vi "Stroke Calibration Report.vi"(8 "error in (no error)":errorcluster, 9 "measured_value":dbl, 10 "operator_name":string="Kiran", 11 "Instrument_serial Number":string="021099") -> (0 "error out":errorcluster, 3 "return value":string)   [LabVIEW 2025]
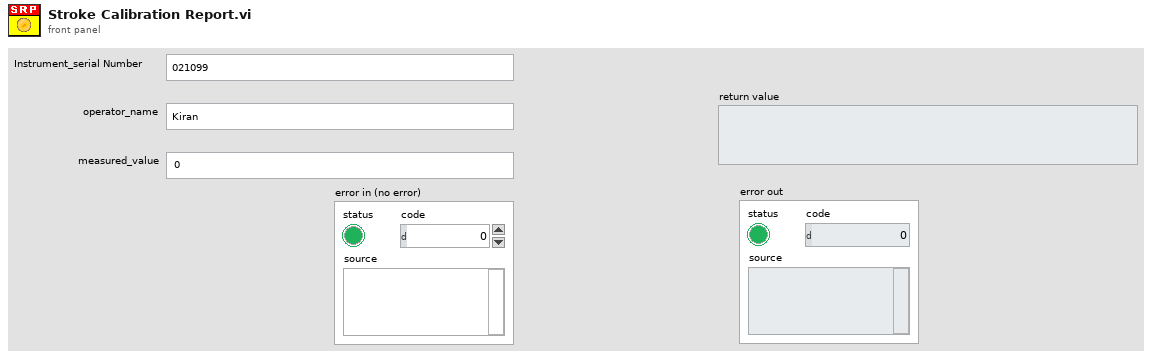
[diagram p1: front panel]
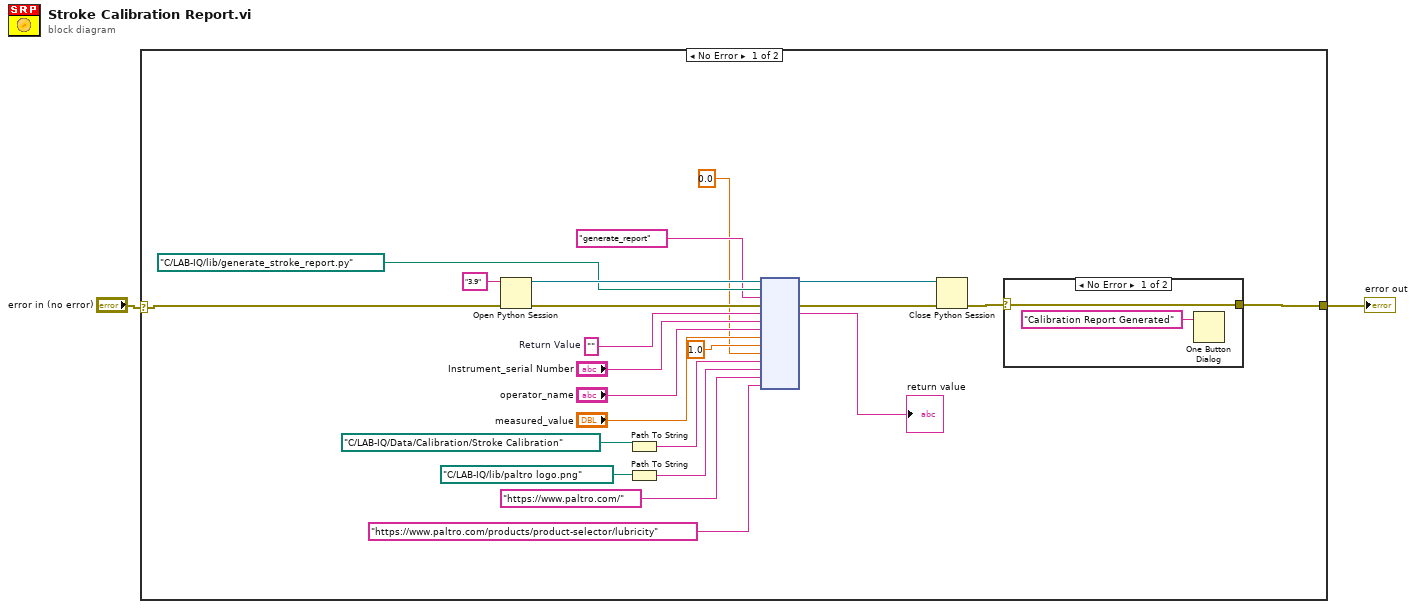
[diagram p0: block diagram]
diagram:
  n1 = case shown="No Error" "error in (no error)" {
    selector: "error in (no error)" -> [w5 _]
    tunnel: [w3 _] -> w2
    frame No Error {
      w20 = ""  # Return Value
      n2 = Open Python Session(python version="3.9" ("Python version"), 3:w5) -> (session out=w24:refnum<k35>, error out=w23:errorcluster)  [unwired: 1 in]
      n3 = Path To String(path=path "C:/LAB-IQ/Data/Calibration/Stroke Calibration" ("output_dir")) -> (string=w8:string)
      n4 = Path To String(path=path "C:/LAB-IQ/lib/paltro logo.png" ("logo_path")) -> (string=w9:string)
      n5 = node(w24, path "C:/LAB-IQ/lib/generate_stroke_report.py" ("Python path"), "generate_report" ("function name"), w23, w20, "Instrument_serial Number", "operator_name", "measured_value", 1.0 ("measured_value"), 0.0 ("measured_value"), w8, w9, "https://www.paltro.com/" ("logo_link_url"), "https://www.paltro.com/products/product-selector/lubricity" ("footer_link_url")) -> (w12:refnum<k35>, w13:errorcluster, →"return value":string)  [unwired: 9 in, 2 out]
      n6 = Close Python Session(session in=w12, error in=w13) -> (11:w4:errorcluster)
      n7 = case shown="No Error" w4 {
        selector: w4 -> [w27 _]
        tunnel: [w27 _] -> w3
        frame No Error {
          n8 = One Button Dialog(message="Calibration Report Generated") -> ()  [unwired: 1 in, 1 out]
        }
        frame Error {
        }
      }
    }
    frame Error {
    }
  }
  "error out" <- w2
